vi "VI_SALTO.vi"(0 "reference":refnum<vi>) -> ()   [LabVIEW 2017]
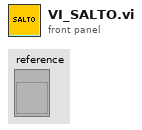
[diagram p1: front panel]
types:
  T1 = enum32{"Bad", "Idle", "Run top level", "Running"}
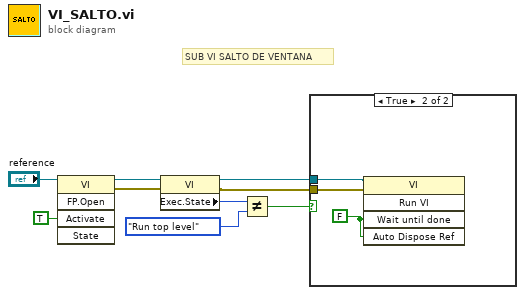
[diagram p0: block diagram]
diagram:
  # "SUB VI SALTO DE VENTANA"
  n1 = invoke class="VI" method="FP.Open"(reference="reference", "Activate"=TRUE ("Activate?")) -> (reference out=w6:refnum<vi>, error out=w5:errorcluster)  [unwired: 3 in, 3 out]
  n2 = property class="VI"(reference=w6, error in=w5) -> (reference out=w8:refnum<vi>, error out=w7:errorcluster, "Exec.State"=w9:T1)
  n3 = Not Equal?(x=w9, y=T1."Run top level") -> (x != y?=w1:bool)
  n4 = case shown="True" w1 {
    tunnel: w8 -> [_ w11]
    tunnel: w7 -> [_ w10]
    frame False {
    }
    frame True {
      w12 = FALSE ("Wait Until Done")
      n5 = invoke class="VI" method="Run VI"(reference=w11, error in=w10, "Wait until done"=w12, "Auto Dispose Ref"=w12) -> ()  [unwired: 1 in, 5 out]
    }
  }
